vi "Data_File_Init RLT.vi"(0 "Data Directory In:":path=path "c:/data", 5 "Ambient Temp,RH:":string="068,50", 7 "Version In:":string="DGnn", 9 "Computer Name In:":string="7A", 11 "error in (no error)":errorcluster, 12 "File Extension:":string="csv") -> (4 "FileNameA":path caption="FileName", 6 "FileNameB":path caption="FileName", 8 "FileNameC":path caption="FileName", 10 "FileNameD":path caption="FileName", 15 "error out":errorcluster)   [LabVIEW 2011]
uses:
  Global HEWH.vi
  <vilib>/Utility/file.llb/Write To Spreadsheet File (string).vi
panel:
  in  "Mode A:":string(combo)
  in  "Mode D:":string(combo)
  in  "Mode C:":string(combo)
  in  "Mode B:":string(combo)
  in  "Unit D:":string
  in  "Comments D:":string="R134A Charge Level: 50g"
  in  "Station D:":string="1A"
  in  "Model D:":string="DC BUILD"
  in  "Unit C:":string
  in  "Comments C:":string="R134A Charge Level: 50g"
  in  "Station C:":string="1A"
  in  "Model C:":string="DC BUILD"
  in  "Unit B:":string
  in  "Comments B:":string="R134A Charge Level: 50g"
  in  "Station B:":string="1A"
  in  "Model B:":string="DC BUILD"
  out "Computer:":string="1A"
  in  "TR Number:":string
  in  "Test Number:":i32 format="%03.0f"
  in  "Unit A:":string
  in  "stop":bool
  in  "Comments A:":string="R134A Charge Level: 50g"
  in  "Technician:":string="JYC"
  in  "Engineer:":string="JYC"
  in  "Test_Title:":string="RLT"
  in  "Station A:":string="1A"
  out "Version:":string="DGnn"
  out "Ambient Temp,RH In:":string="HeatUP"
  out "Date:":string="DGnn"
  in  "Model A:":string="DC BUILD"
  # "yyyymmdd_hhmm_ttttt_uuuuu_nnn_xx_ppp_Trrrrrrrr\nWhere:\nyyyymmdd - day, month as 3 chars, 4 digit year(automatic)\nhhmm - hour and minute (24 hr) test started (automatic)\nttttt - test type name, (automatic)\nuuuuu - is unit number\nnnn - First 3 chars of Ambient Temp/RH\nxx - Mode (HY, SE, EH, HD)\nppp - Test Station\nTrrrrrrrr - 8 digit TR #"
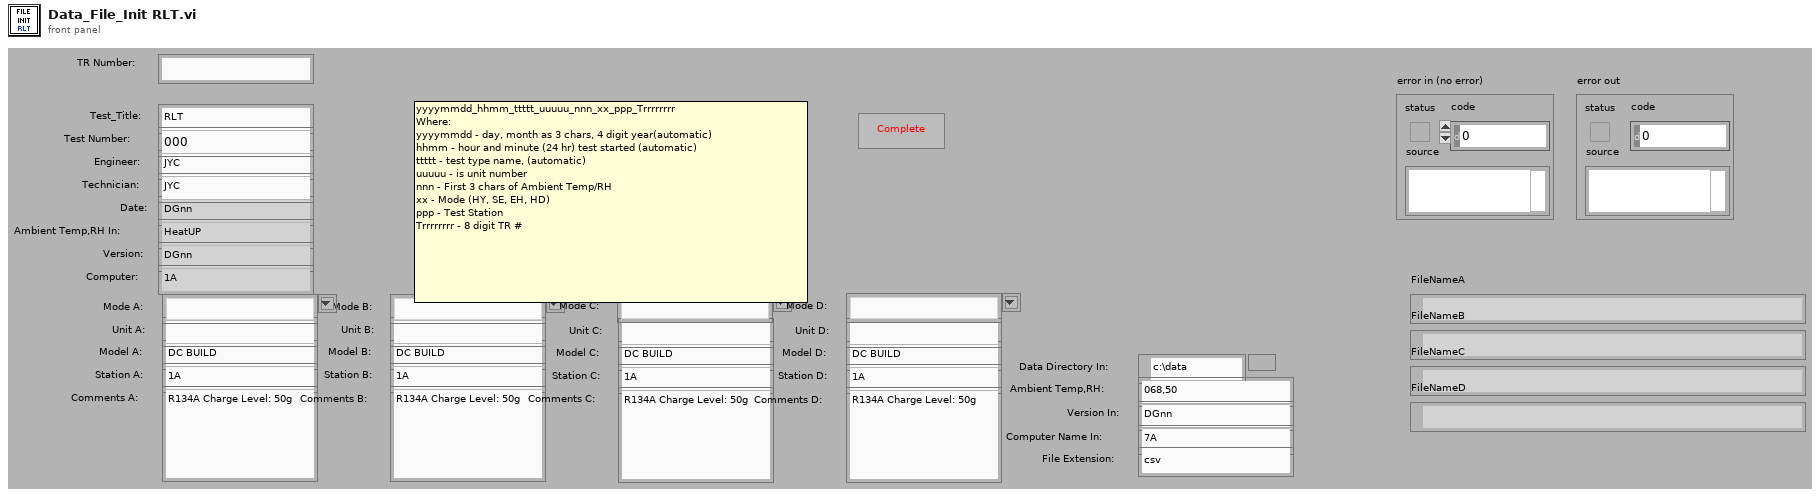
[diagram p1: front panel]
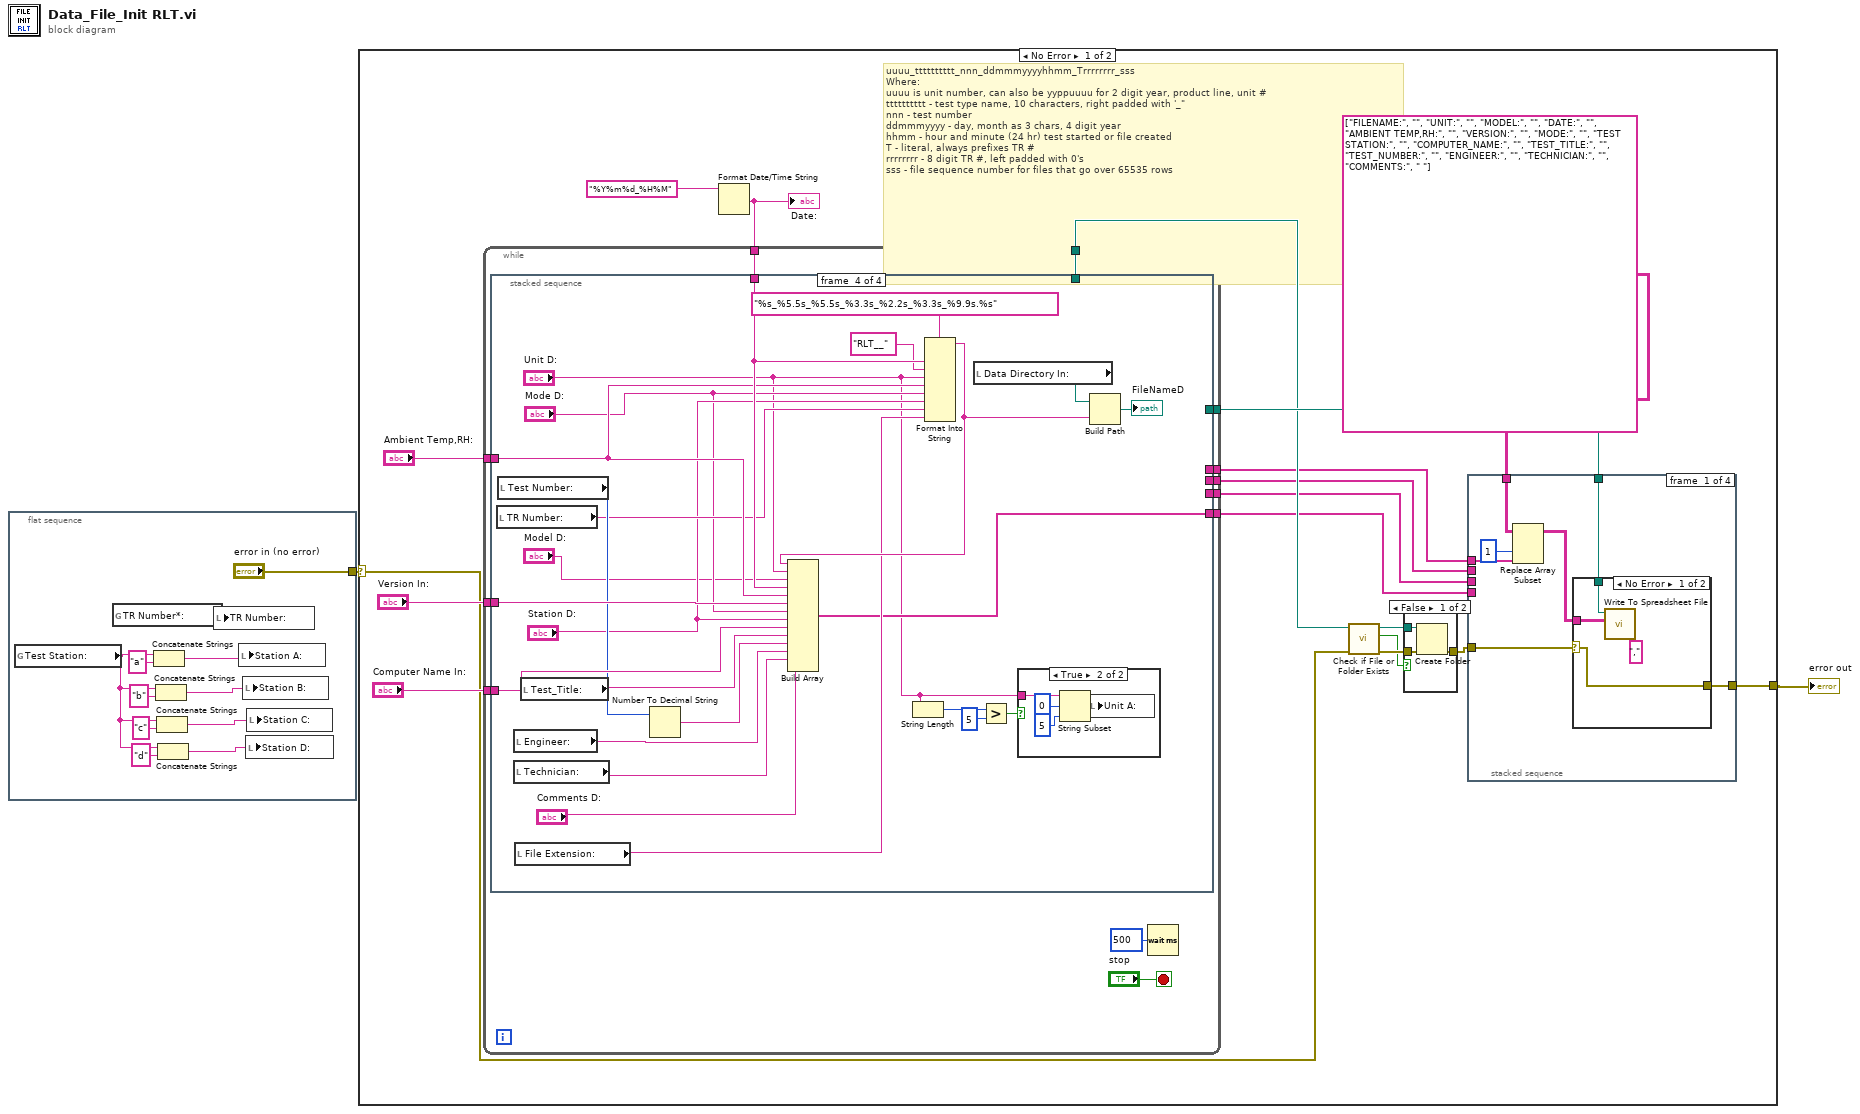
[diagram p0: block diagram]
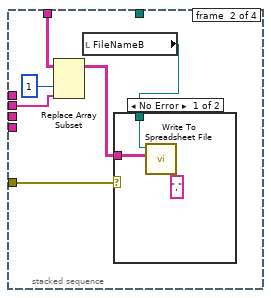
[diagram p3: hidden frame]
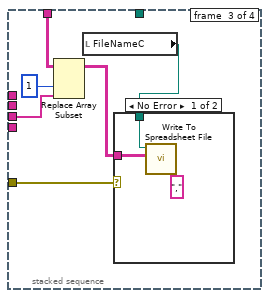
[diagram p5: hidden frame]
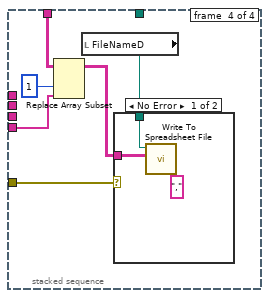
[diagram p7: hidden frame]
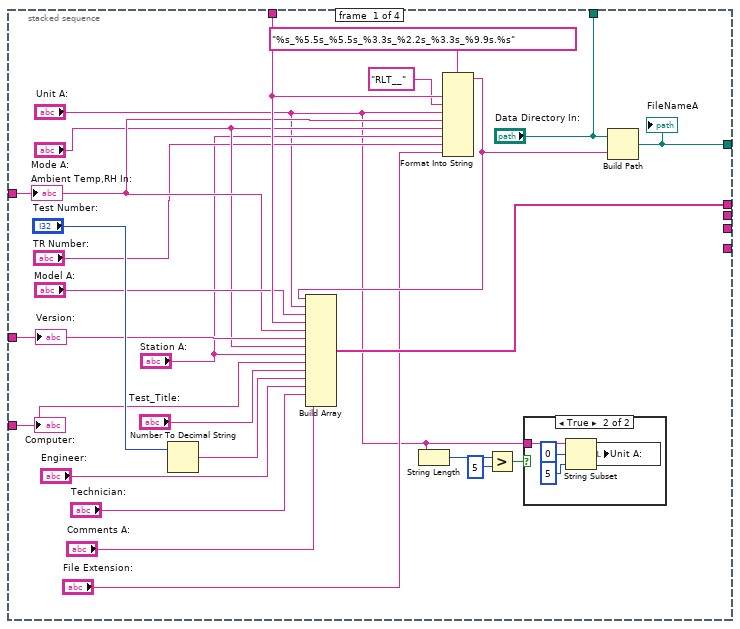
[diagram p10: hidden frame]
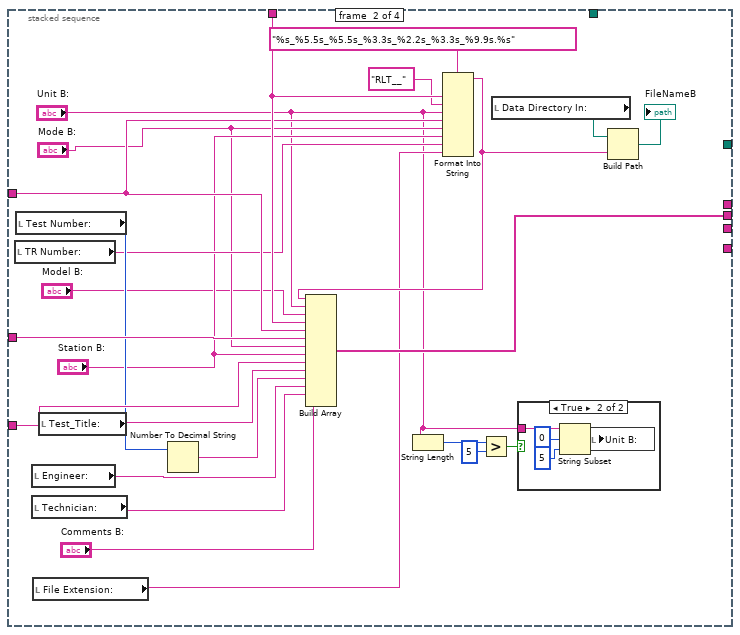
[diagram p12: hidden frame]
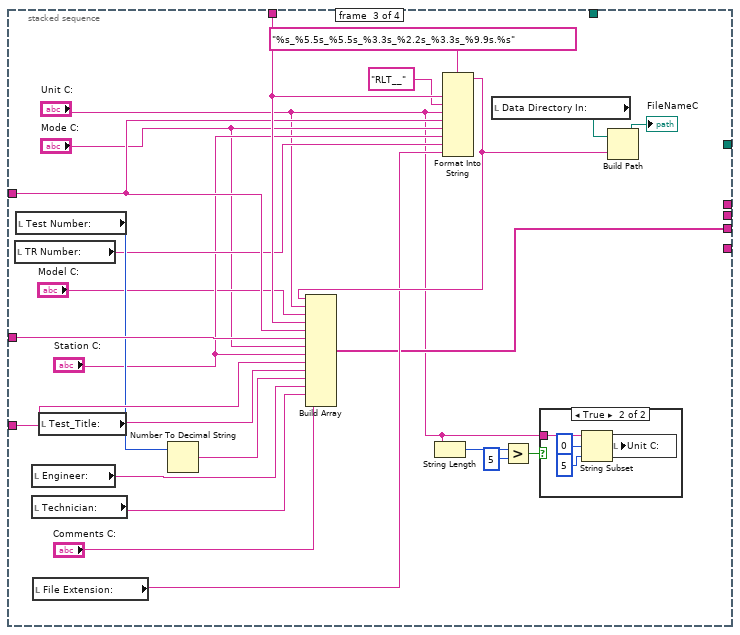
[diagram p14: hidden frame]
diagram:
  n1 = flat-sequence {
    tunnel: ["error in (no error)"] -> w1
    frame #0 {
      n2 = global read "Global HEWH.vi" "Test Station:"() -> (w12:string)
      n3 = global read "Global HEWH.vi" "TR Number*:"() -> (w11:string)
      n4 = Concatenate Strings(w12, "a" ("string")) -> (w10:string)
      n5 = Concatenate Strings(w12, "b" ("string")) -> (w8:string)
      n6 = Concatenate Strings(w12, "c" ("string")) -> (w6:string)
      n7 = Concatenate Strings(w12, "d" ("string")) -> (w4:string)
      n8 = local write "TR Number:"(w11) -> ()
      n9 = local write "Station A:"(w10) -> ()
      n10 = local write "Station B:"(w8) -> ()
      n11 = local write "Station D:"(w4) -> ()
      n12 = local write "Station C:"(w6) -> ()
    }
  }
  n13 = case shown="No Error" w1 {
    selector: w1 -> [w15 w203]
    tunnel: [w27 w203] -> w2
    frame No Error {
      # "uuuu_tttttttttt_nnn_ddmmmyyyyhhmm_Trrrrrrrr_sss\nWhere:\nuuuu is unit number, can also be yyppuuuu for 2 digit year, product line, unit #\ntttttttttt - test type name, 10 characters, right padded with '_\"\nnnn - test number\nddmmmyyyy - day, month as 3 chars, 4 digit year\nhhmm - hour and minute (24 hr) test started or file created\nT - literal, always prefixes TR #\nrrrrrrrr - 8 digit TR #, left padded with 0's\nsss - file sequence number for files that go over 65535 rows"
      n14 = Format Date/Time String(time format string (%c)="%Y%m%d_%H%M") -> (date/time string=w31:string)  [unwired: 2 out]
      "Date:" <- w31
      n15 = while {
        tunnel: w31 -> [w83]
        tunnel: [w78] -> w20
        tunnel: [w85] -> w26
        tunnel: [w84] -> w25
        tunnel: "Ambient Temp,RH:" -> [w81]
        tunnel: "Version In:" -> [w80]
        tunnel: "Computer Name In:" -> [w79]
        tunnel: [w77] -> w19
        tunnel: [w76] -> w18
        tunnel: [w75] -> w16
        stop <- "stop" stop-if-true
        n16 = stacked-sequence {
          tunnel: [w106 _ _ _] -> w85
          tunnel: ["Data Directory In:" _ _ _] -> w84
          tunnel: w83 -> [w99 w136 w165 w194]
          tunnel: w81 -> [w96 w134 w163 w192]
          tunnel: w80 -> [w104 w139 w168 w197]
          tunnel: w79 -> [w92 w133 w162 w191]
          tunnel: [w102 _ _ _] -> w78
          tunnel: [_ w130 _ _] -> w77
          tunnel: [_ _ w154 _] -> w76
          tunnel: [_ _ _ w183] -> w75
          frame #0 {
            n17 = Number To Decimal String(number="Test Number:") -> (decimal integer string=w110:string)  [unwired: 1 in]
            n18 = String Length(string="Unit A:") -> (length=w90:i32)
            n19 = Format Into String(format string="%s_%5.5s_%5.5s_%3.3s_%2.2s_%3.3s_%9.9s.%s", w99, "RLT__" ("input 2"), "Unit A:", w96, "Mode A:", "Station A:", "TR Number:", "File Extension:") -> (resulting string=w100:string)  [unwired: 2 in, 1 out]
            n20 = Build Array(w100, "Unit A:", "Model A:", w99, w96, w104, "Mode A:", "Station A:", w92, "Test_Title:", w110, "Engineer:", "Technician:", "Comments A:") -> (w102:string[])
            n21 = Greater?(x=w90, y=5) -> (0:w88:bool)
            n22 = case shown="True" w88 {
              tunnel: "Unit A:" -> [_ w115]
              frame False {
              }
              frame True {
                n23 = String Subset(string=w115, offset (0)=0, length (rest)=5 ("length (rest)")) -> (substring=w112:string)
                n24 = local write "Unit A:"(w112) -> ()
              }
            }
            n25 = Build Path(base path="Data Directory In:", name or relative path=w100) -> (appended path=w106:path)
            "FileNameA" <- w106
            "Ambient Temp,RH In:" <- w96
            "Version:" <- w104
            "Computer:" <- w92
          }
          frame #1 {
            n26 = local read "TR Number:"() -> (w128:string)
            n27 = local read "Test Number:"() -> (w129:i32)
            n28 = local read "Engineer:"() -> (w125:string)
            n29 = local read "Technician:"() -> (w124:string)
            n30 = local read "File Extension:"() -> (w122:string)
            n31 = local read "Test_Title:"() -> (w126:string)
            n32 = Number To Decimal String(number=w129) -> (decimal integer string=w140:string)  [unwired: 1 in]
            n33 = String Length(string="Unit B:") -> (length=w119:i32)
            n34 = Format Into String(format string="%s_%5.5s_%5.5s_%3.3s_%2.2s_%3.3s_%9.9s.%s", w136, "RLT__" ("input 2"), "Unit B:", w134, "Mode B:", "Station B:", w128, w122) -> (resulting string=w137:string)  [unwired: 2 in, 1 out]
            n35 = Build Array(w137, "Unit B:", "Model B:", w136, w134, w139, "Mode B:", "Station B:", w133, w126, w140, w125, w124, "Comments B:") -> (w130:string[])
            n36 = Greater?(x=w119, y=5) -> (0:w117:bool)
            n37 = local read "Data Directory In:"() -> (w131:path)
            n38 = case shown="True" w117 {
              tunnel: "Unit B:" -> [_ w144]
              frame False {
              }
              frame True {
                n39 = String Subset(string=w144, offset (0)=0, length (rest)=5 ("length (rest)")) -> (substring=w141:string)
                n40 = local write "Unit B:"(w141) -> ()
              }
            }
            n41 = Build Path(base path=w131, name or relative path=w137) -> (appended path=→"FileNameB":path)
          }
          frame #2 {
            n42 = local read "TR Number:"() -> (w159:string)
            n43 = local read "Test Number:"() -> (w160:i32)
            n44 = local read "Engineer:"() -> (w157:string)
            n45 = local read "Technician:"() -> (w156:string)
            n46 = local read "File Extension:"() -> (w155:string)
            n47 = local read "Test_Title:"() -> (w158:string)
            n48 = Number To Decimal String(number=w160) -> (decimal integer string=w169:string)  [unwired: 1 in]
            n49 = String Length(string="Unit C:") -> (length=w148:i32)
            n50 = Format Into String(format string="%s_%5.5s_%5.5s_%3.3s_%2.2s_%3.3s_%9.9s.%s", w165, "RLT__" ("input 2"), "Unit C:", w163, "Mode C:", "Station C:", w159, w155) -> (resulting string=w166:string)  [unwired: 2 in, 1 out]
            n51 = Build Array(w166, "Unit C:", "Model C:", w165, w163, w168, "Mode C:", "Station C:", w162, w158, w169, w157, w156, "Comments C:") -> (w154:string[])
            n52 = local read "Data Directory In:"() -> (w161:path)
            n53 = Greater?(x=w148, y=5) -> (0:w146:bool)
            n54 = case shown="True" w146 {
              tunnel: "Unit C:" -> [_ w173]
              frame False {
              }
              frame True {
                n55 = String Subset(string=w173, offset (0)=0, length (rest)=5 ("length (rest)")) -> (substring=w170:string)
                n56 = local write "Unit C:"(w170) -> ()
              }
            }
            n57 = Build Path(base path=w161, name or relative path=w166) -> (appended path=→"FileNameC":path)
          }
          frame #3 {
            n58 = local read "TR Number:"() -> (w188:string)
            n59 = local read "Test Number:"() -> (w189:i32)
            n60 = local read "Engineer:"() -> (w186:string)
            n61 = local read "Technician:"() -> (w185:string)
            n62 = local read "File Extension:"() -> (w184:string)
            n63 = local read "Test_Title:"() -> (w187:string)
            n64 = Number To Decimal String(number=w189) -> (decimal integer string=w198:string)  [unwired: 1 in]
            n65 = String Length(string="Unit D:") -> (length=w177:i32)
            n66 = Format Into String(format string="%s_%5.5s_%5.5s_%3.3s_%2.2s_%3.3s_%9.9s.%s", w194, "RLT__" ("input 2"), "Unit D:", w192, "Mode D:", "Station D:", w188, w184) -> (resulting string=w195:string)  [unwired: 2 in, 1 out]
            n67 = Build Array(w195, "Unit D:", "Model D:", w194, w192, w197, "Mode D:", "Station D:", w191, w187, w198, w186, w185, "Comments D:") -> (w183:string[])
            n68 = local read "Data Directory In:"() -> (w190:path)
            n69 = Greater?(x=w177, y=5) -> (0:w175:bool)
            n70 = case shown="True" w175 {
              tunnel: "Unit D:" -> [_ w202]
              frame False {
              }
              frame True {
                n71 = String Subset(string=w202, offset (0)=0, length (rest)=5 ("length (rest)")) -> (substring=w199:string)
                n72 = local write "Unit A:"(w199) -> ()
              }
            }
            n73 = Build Path(base path=w190, name or relative path=w195) -> (appended path=→"FileNameD":path)
          }
        }
        n74 = Wait (ms)(milliseconds to wait=u32 500) -> ()  [unwired: 1 out]
      }
      n75 = call <vilib>:"Check if File or Folder Exists.vi"("error in (no error)"=w15, "path"=w25) -> ("error out"=w30:errorcluster, "file or folder exists?"=w28:bool, "dup path"=w29:path)  [unwired: 7 out]
      n76 = case shown="False" w28 {
        tunnel: w29 -> [w71 _]
        tunnel: w30 -> [w73 w74]
        tunnel: [w72 w74] -> w17
        frame False {
          n77 = Create Folder(path (use dialog)=w71, error in=w73) -> (error out=w72:errorcluster)  [unwired: 3 out]
        }
        frame True {
        }
      }
      n78 = stacked-sequence {
        tunnel: w17 -> [w38 w44 w53 w63]
        tunnel: [w32 _ _ _] -> w27
        tunnel: w26 -> [w37 _ _ _]
        tunnel: string[][] [["FILENAME:", ""], ["UNIT:", ""], ["MODEL:", ""], ["DATE:", ""], ["AMBIENT TEMP,RH:", ""], ["VERSION:", ""], ["MODE:", ""], ["TEST STATION:", ""], ["COMPUTER_NAME:", ""], ["TEST_TITLE:", ""], ["TEST_NUMBER:", ""], ["ENGINEER:", ""], ["TECHNICIAN:", ""], ["COMMENTS:", " "]] ("array") -> [w34 w47 w56 w65]
        tunnel: w20 -> [w33 _ _ _]
        tunnel: w19 -> [_ w45 _ _]
        tunnel: w18 -> [_ _ w54 _]
        tunnel: w16 -> [_ _ _ w62]
        frame #0 {
          n79 = Replace Array Subset(array=w34, new element=w33, index (col)=1 ("disabled index (col)")) -> (w35:string[][])  [unwired: 1 in]
          n80 = case shown="No Error" w38 {
            selector: w38 -> [w40 w43]
            tunnel: w35 -> [w42 _]
            tunnel: [w40 w43] -> w32
            tunnel: w37 -> [w39 _]
            frame No Error {
              n81 = call-poly <vilib>:"Write To Spreadsheet File.vi"("delimiter (\\t)"="," ("delimiter (\\t)"), "2D data"=w42, "file path (dialog if empty)"=w39) -> ()  [unwired: 5 in, 1 out]
            }
            frame Error {
            }
          }
        }
        frame #1 {
          n82 = Replace Array Subset(array=w47, new element=w45, index (col)=1 ("disabled index (col)")) -> (w48:string[][])  [unwired: 1 in]
          n83 = local read "FileNameB"() -> (w46:path)
          n84 = case shown="No Error" w44 {
            tunnel: w48 -> [w52 _]
            tunnel: w46 -> [w50 _]
            frame No Error {
              n85 = call-poly <vilib>:"Write To Spreadsheet File.vi"("delimiter (\\t)"="," ("delimiter (\\t)"), "2D data"=w52, "file path (dialog if empty)"=w50) -> ()  [unwired: 5 in, 1 out]
            }
            frame Error {
            }
          }
        }
        frame #2 {
          n86 = Replace Array Subset(array=w56, new element=w54, index (col)=1 ("disabled index (col)")) -> (w57:string[][])  [unwired: 1 in]
          n87 = local read "FileNameC"() -> (w55:path)
          n88 = case shown="No Error" w53 {
            tunnel: w57 -> [w61 _]
            tunnel: w55 -> [w59 _]
            frame No Error {
              n89 = call-poly <vilib>:"Write To Spreadsheet File.vi"("delimiter (\\t)"="," ("delimiter (\\t)"), "2D data"=w61, "file path (dialog if empty)"=w59) -> ()  [unwired: 5 in, 1 out]
            }
            frame Error {
            }
          }
        }
        frame #3 {
          n90 = Replace Array Subset(array=w65, new element=w62, index (col)=1 ("disabled index (col)")) -> (w66:string[][])  [unwired: 1 in]
          n91 = local read "FileNameD"() -> (w64:path)
          n92 = case shown="No Error" w63 {
            tunnel: w66 -> [w70 _]
            tunnel: w64 -> [w68 _]
            frame No Error {
              n93 = call-poly <vilib>:"Write To Spreadsheet File.vi"("delimiter (\\t)"="," ("delimiter (\\t)"), "2D data"=w70, "file path (dialog if empty)"=w68) -> ()  [unwired: 5 in, 1 out]
            }
            frame Error {
            }
          }
        }
      }
    }
    frame Error {
    }
  }
  "error out" <- w2
